vi "getT7Inclinometer.vi"(11 "Model in":refnum<class "Model.lvclass">) -> (2 "T7Inclinometer":refnum<class "T7Inclinometer.lvclass">, 3 "Model out":refnum<class "Model.lvclass">)   [LabVIEW 2016, in "Model.lvclass"]
uses:
  Model.lvclass
  Common_RT_T7Inclinometer/T7Inclinometer/T7Inclinometer.lvclass
  Model.lvclass/Model.ctl
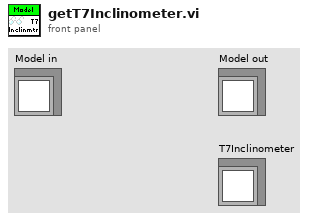
[diagram p1: front panel]
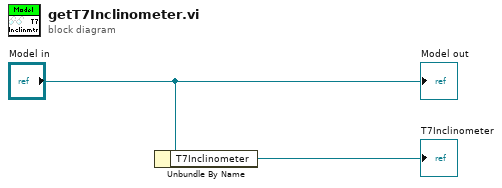
[diagram p0: block diagram]
diagram:
  n1 = Unbundle By Name("Model in") -> ("T7Inclinometer"=→"T7Inclinometer":refnum<class "T7Inclinometer.lvclass">)
  "Model out" <- "Model in"
